vi "ISEG_HVSystemGUI.panel.vi"(0 "object ref":refnum<vi>, 5 "error in (no error)":errorcluster) -> (19 "error out":errorcluster)   [LabVIEW 2014, in "ISEG_HVSystemGUI.lvlib"]
doc: "This is just an example for a ISEG HV System GUI .\n\nLicense Agreement for this software:\n\nCopyright (C)\nGesellschaft für Schwerionenforschung, GSI\nPlanckstr. 1\n64291 Darmstadt\nGermany\n\nContact: D.Beck@gsi.de \n\nThis program is free software; you can redistribute it and/or modify it under the terms of the GNU General Public License as published by the Free Software Foundation; either version 2 of the license, or (at your option) any later version.\n\nThis program is distributed in the hope that it will be useful, but WITHOUT ANYW ARRANTY; without even the implied warranty of MERCHANTABILITY or FITNESS FOR A PARTICULAR PURPOSE. See the GNU General License for more details (http://www.gnu.org).\n\nGesellschaft für Schwerionenforschung, GSI\nPlanckstr. 1, 64291 Darmstadt, Germany\nFor all questions and ideas contact: M.Richter@gsi.de, H.Brand@gsi.de or D.Beck@gsi.de.\nLast update: 18-DEC-2002"
uses:
  ISEG_HVSystemGUI.lvlib
  CSlibraries-extern/DimLVEvent/DimIndicators/DimIndicators.anyType.ctl
  CSlibraries-extern/DimLVEvent/DimIndicators/DimIndicators.numericType.ctl
  CS_Core/CSSystem/CoreDefs/CoreDefs.call_type.ctl
  CS_Core/BaseProcess/BaseProcess.descriptor string definition.ctl
  CS_Core/CSSystem/CoreDefs/CoreDefs.rawDataType.ctl
  CS_Core/CSSystem/CoreLib/CoreLib.short 2 byte array.vi
  CS_Core/CSSystem/CoreLib/CoreLib.double 2 byte array.vi
  CS_Core/CSSystem/CoreLib/CoreLib.string 2 byte array.vi
  CSlibraries/UtilityLib/UtilityLib.lvlib
  CS_Core/CSSystem/CoreLib/CoreLib.lvlib
  CSlibraries-extern/DimLVEvent/DimIndicators/DimIndicators.lvlib
  CS_Core/CSSystem/CSSystemLib/CSSystemLib.lvlib
  CS_Core/BaseProcess/BaseProcess.lvlib
panel:
  in  "Refresh":T1
  in  "Force":T2
  in  "Mode1/Mode2":bool caption="Status_Force"
  in  "Refresh":dbl
  in  "Connected":T2
  in  "Active":T2
  out "Connected":bool
  out "Active":bool
  in  "call cluster in":T3={"Object"="", "Selector"="", "CallType"=enum."synchronous", "Async Object"="", "Async Selector"="", "Data Descriptor"="", "Data"=[], "Error #"=0, "Expire"=0}
  in  "DeviceState":T1
  out "Object Name":string
  in  "Pr ID":T2
  in  "OPC Version":T2
  in  "CAN":T2
  in  "Open BoardGUI":bool
  in  "Board":i16
  in  "stop":bool
  out "Pr ID":string
  out "OPC Version":string
  out "CAN":string caption="Status_CAN bus"
  out "loop counter":i32
  out "time stamp":timestamp
  # ":"
  # "Mode 2"
  # "Mode1"
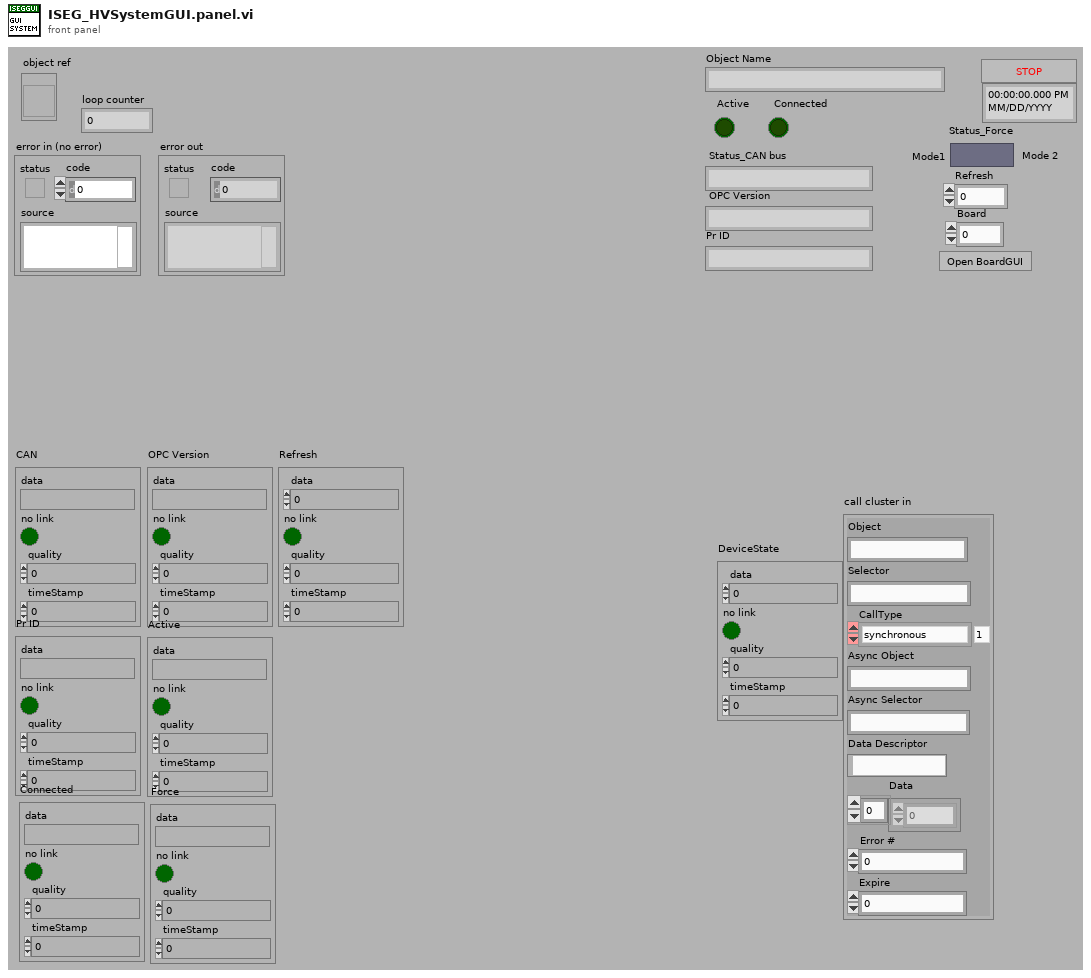
[diagram p1: front panel]
types:
  T1 = typedef "DimIndicators.lvlib/DimIndicators.numericType.ctl" = cluster{"data":dbl, "no link":bool, "quality":i32, "timeStamp":dbl}
  T2 = typedef "DimIndicators.lvlib/DimIndicators.anyType.ctl" = cluster{"data":string, "no link":bool, "quality":i32, "timeStamp":dbl}
  T3 = typedef "CoreDefs.call_type.ctl" = cluster{"Object":string, "Selector":string, "CallType":enum16{"simple", "synchronous", "asynchronous"}, "Async Object":string, "Async Selector":string, "Data Descriptor":T4, "Data":T5, "Error #":i32, "Expire":u32}
  T4 = typedef "BaseProcess.lvlib/BaseProcess.descriptor string definition.ctl" = string
  T5 = typedef "CoreDefs.rawDataType.ctl" = i8[]
  T6 = typedef "ISEG_HVSystemGUI.lvlib/ISEG_HVSystemGUI.i attribute.ctl" = cluster{"System Name":string, "Object Name":string, "Prefix":string}
  T7 = typedef "UtilityLib.lvlib/UtilityLib.valueStatus.ctl" = enum16{"no info available", "stand by/off", "on", "warning", "alarm/malfunction", "not implemented", "user action required", "important information", "system default", "control default", "indicator default", "button default"}
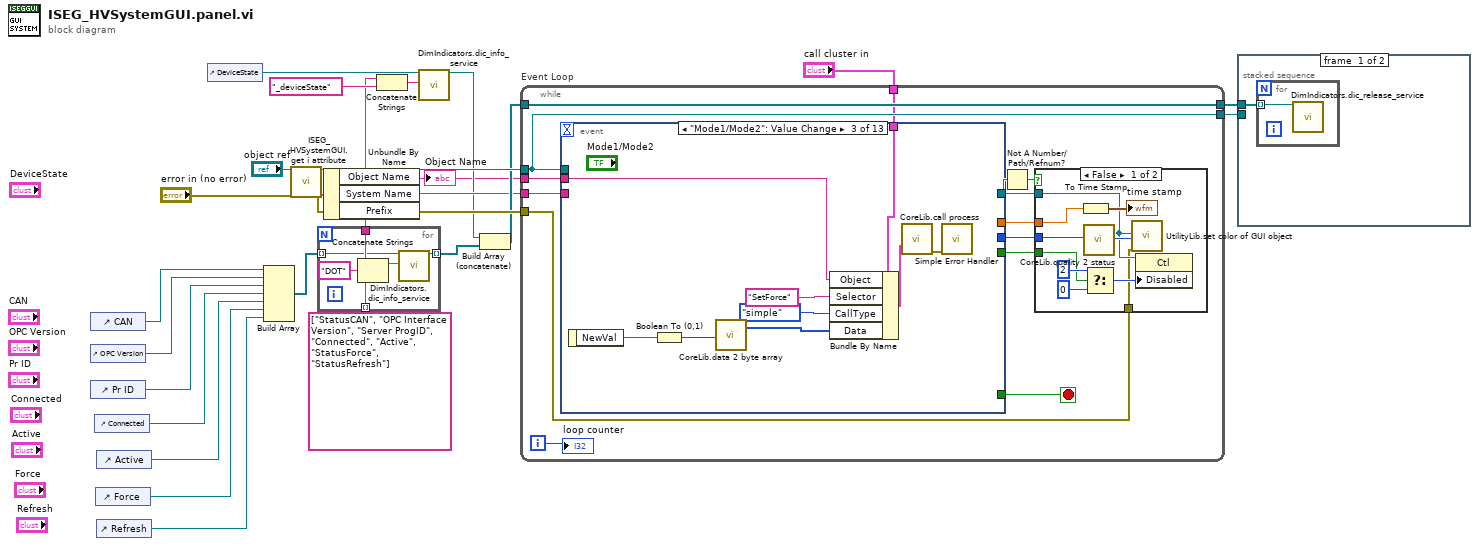
[diagram p0: block diagram]
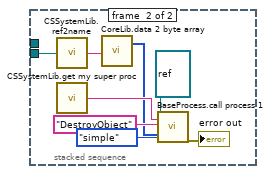
[diagram p2: hidden frame]
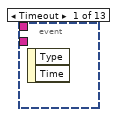
[diagram p4: hidden frame]
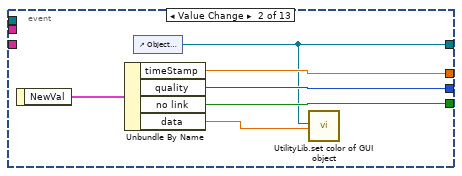
[diagram p5: hidden frame]
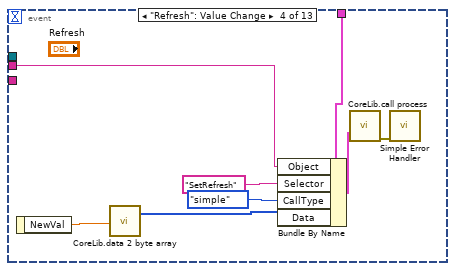
[diagram p6: hidden frame]
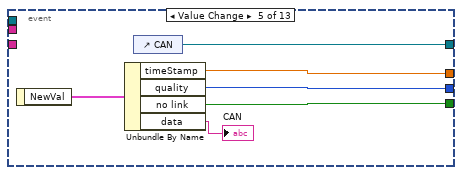
[diagram p7: hidden frame]
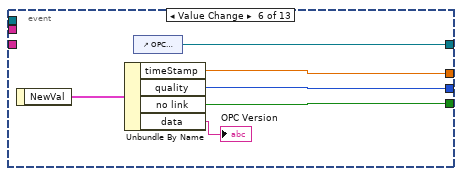
[diagram p8: hidden frame]
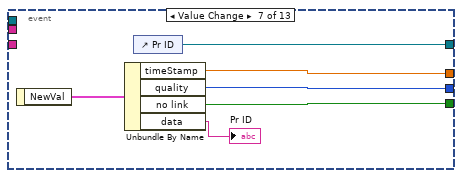
[diagram p9: hidden frame]
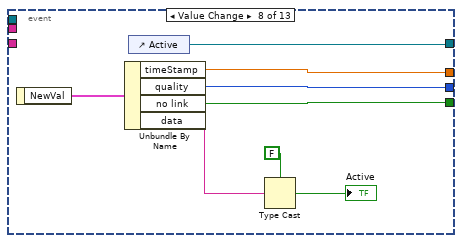
[diagram p10: hidden frame]
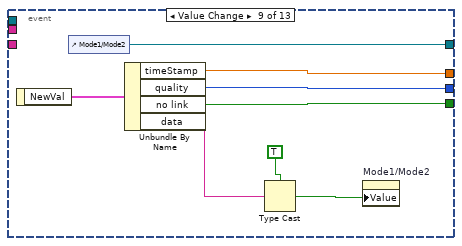
[diagram p11: hidden frame]
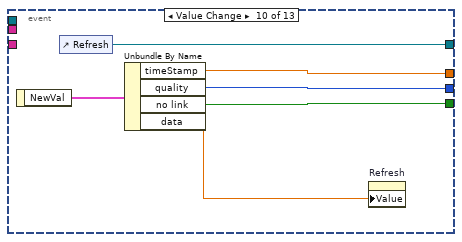
[diagram p12: hidden frame]
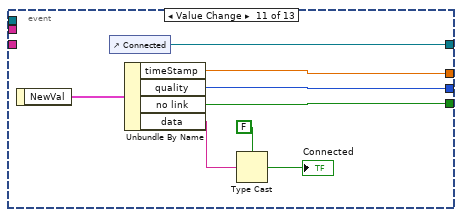
[diagram p13: hidden frame]
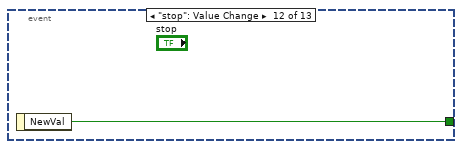
[diagram p14: hidden frame]
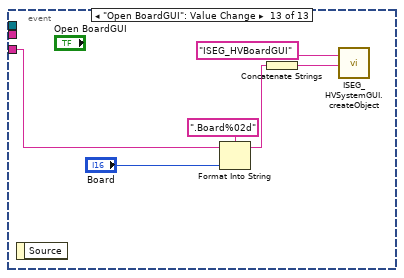
[diagram p15: hidden frame]
diagram:
  n1 = control-ref of="CAN"() -> (w9:refnum<vi>)
  n2 = control-ref of="OPC Version"() -> (w8:refnum<vi>)
  n3 = control-ref of="Pr ID"() -> (w7:refnum<vi>)
  n4 = control-ref of="Connected"() -> (w3:refnum<vi>)
  n5 = control-ref of="Force"() -> (w2:refnum<vi>)
  n6 = control-ref of="Active"() -> (w4:refnum<vi>)
  n7 = control-ref of="Refresh"() -> (w1:refnum<vi>)
  n8 = control-ref of="DeviceState"() -> (w12:refnum<vi>)
  n9 = Build Array(w9, w8, w7, w3, w4, w2, w1) -> (w21:refnum<vi>[])
  n10 = call "ISEG_HVSystemGUI.get i attribute.vi"("i ref in"="object ref", "error in (no error)"="error in (no error)") -> ("i ref out"=w24:refnum<vi>, "i attribute"=w23:T6, "error out"=w18:errorcluster)  [unwired: 15 in]
  n11 = Unbundle By Name(w23) -> ("Object Name"=w11:string, "System Name"=w16:string, "Prefix"=w5:string)
  "Object Name" <- w11
  n12 = for {
    tunnel: w5 -> [w31]
    tunnel: string[] ["StatusCAN", "OPC Interface Version", "Server ProgID", "Connected", "Active", "StatusForce", "StatusRefresh"] ("Properties") -> [w30] mode=indexing
    tunnel: w21 -> [w28] mode=indexing
    tunnel: [w27] -> w6 mode=indexing
    n13 = Concatenate Strings(w31, "DOT" ("string"), w30) -> (w29:string)
    n14 = call "DimIndicators.dic_info_service.vi"("controlRef"=w28, "serviceName"=w29) -> ("controlRef out"=w27:refnum<vi>)  [unwired: 16 in, 1 out]
  }
  n15 = Concatenate Strings(w11, "_deviceState" ("string")) -> (w14:string)
  n16 = call "DimIndicators.dic_info_service.vi"("controlRef"=w12, "serviceName"=w14) -> ("controlRef out"=w13:refnum<vi>)  [unwired: 16 in, 1 out]
  n17 = Build Array (concatenate)(w13, w6) -> (w17:refnum<vi>[])
  n18 = while "Event Loop" {
    tunnel: w24 -> [w43]
    tunnel: [w43] -> w26
    tunnel: [w42] -> w20
    tunnel: w17 -> [w42]
    tunnel: w18 -> [w39]
    tunnel: w16 -> [w38]
    tunnel: w11 -> [w34]
    tunnel: "call cluster in" -> [w33]
    i -> [w44]
    stop <- w45 stop-if-true
    n19 = event shown="[2] \"Mode1/Mode2\": Value Change" {
      selector: _ -> [_ _ _ _ _ _ _ _ _ _ _ _ _]
      dyn-events: _ -> [_ _ _ _ _ _ _ _ _ _ _ _ _]
      timeout: _ -> [_ _ _ _ _ _ _ _ _ _ _ _ _]
      tunnel: [_ _ _ _ _ _ _ _ _ _ _ w127 _] -> w45
      tunnel: w43 -> [_ _ _ _ _ _ _ _ _ _ _ _ _]
      tunnel: [_ w60 _ _ w84 w90 w96 w104 w112 w118 w126 _ _] -> w41
      tunnel: [_ w59 _ _ w83 w89 w95 w103 w111 w117 w125 _ _] -> w40
      tunnel: [_ w57 _ _ w82 w88 w94 w100 w107 w114 w122 _ _] -> w35
      tunnel: [_ w58 _ _ w81 w87 w93 w102 w110 w116 w124 _ _] -> w37
      tunnel: w38 -> [_ _ _ _ _ _ _ _ _ _ _ _ w133]
      tunnel: w34 -> [_ _ w65 w74 _ _ _ _ _ _ _ _ _]
      tunnel: w33 -> [_ _ w66 w75 _ _ _ _ _ _ _ _ _]
      event Timeout {
        n20 = event-data() -> ()  [unwired: 1 in, 2 out]
      }
      event Value Change {
        n21 = event-data() -> ("NewVal"=w61:T1)  [unwired: 1 in]
        n22 = Unbundle By Name(w61) -> ("timeStamp"=w58:dbl, "quality"=w60:i32, "no link"=w59:bool, "data"=w56:dbl)
        n23 = control-ref of="Object Name"() -> (w57:refnum<vi>)
        n24 = call "UtilityLib.set color of GUI object.vi"("GUI object Ref"=w57, "valueStatus"=w56) -> ()  [unwired: 17 in, 1 out]
      }
      event "Mode1/Mode2": Value Change {
        n25 = event-data() -> ("NewVal"=w67:bool)  [unwired: 1 in]
        n26 = Boolean To (0,1)(Boolean=w67) -> (0, 1=w63:i16)
        n27 = call-poly "CoreLib.data 2 byte array.vi"("i16"=w63) -> ("byteArray out"=w62:T5)  [unwired: 18 in]
        n28 = Bundle By Name(cluster=w66, "Object"=w65, "Selector"="SetForce", "CallType"=enum16{"simple", "synchronous", "asynchronous"}."simple", "Data"=w62) -> (w64:T3)
        n29 = call "CoreLib.call process.vi"("call cluster in"=w64) -> ("error out"=w70:errorcluster)  [unwired: 13 in, 1 out]
        n30 = call <vilib>:"Simple Error Handler.vi"("error in (no error)"=w70) -> ()  [unwired: 4 in, 5 out]
      }
      event "Refresh": Value Change {
        n31 = event-data() -> ("NewVal"=w71:dbl)  [unwired: 1 in]
        n32 = call-poly "CoreLib.data 2 byte array.vi"("f64"=w71) -> ("byteArray out"=w72:T5)  [unwired: 18 in]
        n33 = Bundle By Name(cluster=w75, "Object"=w74, "Selector"="SetRefresh", "CallType"=enum16{"simple", "synchronous", "asynchronous"}."simple", "Data"=w72) -> (w73:T3)
        n34 = call "CoreLib.call process.vi"("call cluster in"=w73) -> ("error out"=w78:errorcluster)  [unwired: 13 in, 1 out]
        n35 = call <vilib>:"Simple Error Handler.vi"("error in (no error)"=w78) -> ()  [unwired: 4 in, 5 out]
      }
      event Value Change {
        n36 = event-data() -> ("NewVal"=w80:T2)  [unwired: 1 in]
        n37 = Unbundle By Name(w80) -> ("timeStamp"=w81:dbl, "quality"=w84:i32, "no link"=w83:bool, "data"=→"CAN":string)
        n38 = control-ref of="CAN"() -> (w82:refnum<vi>)
      }
      event Value Change {
        n39 = event-data() -> ("NewVal"=w86:T2)  [unwired: 1 in]
        n40 = Unbundle By Name(w86) -> ("timeStamp"=w87:dbl, "quality"=w90:i32, "no link"=w89:bool, "data"=→"OPC Version":string)
        n41 = control-ref of="OPC Version"() -> (w88:refnum<vi>)
      }
      event Value Change {
        n42 = event-data() -> ("NewVal"=w92:T2)  [unwired: 1 in]
        n43 = Unbundle By Name(w92) -> ("timeStamp"=w93:dbl, "quality"=w96:i32, "no link"=w95:bool, "data"=→"Pr ID":string)
        n44 = control-ref of="Pr ID"() -> (w94:refnum<vi>)
      }
      event Value Change {
        n45 = event-data() -> ("NewVal"=w101:T2)  [unwired: 1 in]
        n46 = Unbundle By Name(w101) -> ("timeStamp"=w102:dbl, "quality"=w104:i32, "no link"=w103:bool, "data"=w99:string)
        n47 = control-ref of="Active"() -> (w100:refnum<vi>)
        n48 = Type Cast(type=FALSE, x=w99) -> (*(type *) &x=→"Active":bool)
      }
      event Value Change {
        n49 = event-data() -> ("NewVal"=w108:T2)  [unwired: 1 in]
        n50 = control-ref of="Mode1/Mode2"() -> (w107:refnum<vi>)
        n51 = Unbundle By Name(w108) -> ("timeStamp"=w110:dbl, "quality"=w112:i32, "no link"=w111:bool, "data"=w109:string)
        n52 = Type Cast(type=TRUE, x=w109) -> (*(type *) &x=w105:bool)
        n53 = property on="Mode1/Mode2" class="Bool (strict)"("Value"=w105) -> ()  [unwired: 2 in, 2 out]
      }
      event Value Change {
        n54 = event-data() -> ("NewVal"=w115:T1)  [unwired: 1 in]
        n55 = control-ref of="Refresh"() -> (w114:refnum<vi>)
        n56 = Unbundle By Name(w115) -> ("timeStamp"=w116:dbl, "quality"=w118:i32, "no link"=w117:bool, "data"=w113:dbl)
        n57 = property on="Refresh" class="DigNum (strict)"("Value"=w113) -> ()  [unwired: 2 in, 2 out]
      }
      event Value Change {
        n58 = event-data() -> ("NewVal"=w123:T2)  [unwired: 1 in]
        n59 = control-ref of="Connected"() -> (w122:refnum<vi>)
        n60 = Unbundle By Name(w123) -> ("timeStamp"=w124:dbl, "quality"=w126:i32, "no link"=w125:bool, "data"=w119:string)
        n61 = Type Cast(type=FALSE, x=w119) -> (*(type *) &x=→"Connected":bool)
      }
      event "stop": Value Change {
        n62 = event-data() -> ("NewVal"=w127:bool)  [unwired: 1 in]
      }
      event "Open BoardGUI": Value Change {
        n63 = event-data() -> ()  [unwired: 1 in, 1 out]
        n64 = Format Into String(format string=".Board%02d", initial string=w133, "Board") -> (resulting string=w128:string)  [unwired: 1 in, 1 out]
        n65 = Concatenate Strings(w128) -> (w130:string)
        n66 = call "ISEG_HVSystemGUI.createObject.vi"("Class name"="ISEG_HVBoardGUI" ("class name"), "data"=w130) -> ()  [unwired: 17 in, 1 out]
      }
    }
    n67 = Not A Number/Path/Refnum?(number/path/refnum=w35) -> (NaN/Path/Refnum?=w36:bool)
    n68 = case shown="False" w36 {
      tunnel: w41 -> [w52 _]
      tunnel: w40 -> [w51 _]
      tunnel: w35 -> [w47 _]
      tunnel: w37 -> [w49 _]
      tunnel: w39 -> [w46 _]
      frame False {
        n69 = To Time Stamp(1:w49) -> (0:→"time stamp":timestamp)
        n70 = call "CoreLib.quality 2 status.vi"("quality"=w52) -> ("valueStatus"=w48:T7)  [unwired: 18 in]
        n71 = Select(t=u8 2 ("Disabled"), s=w51, f=u8 0) -> (s? t:f=w55:u8)
        n72 = call "UtilityLib.set color of GUI object.vi"("GUI object Ref"=w47, "valueStatus"=w48, "error in (no error)"=w46) -> ()  [unwired: 16 in, 1 out]
        n73 = property class="Ctl"(reference=w47, "Disabled"=w55) -> ()  [unwired: 1 in, 2 out]
      }
      frame True {
      }
    }
    "loop counter" <- w44
  }
  n74 = stacked-sequence {
    tunnel: w26 -> [_ w137]
    tunnel: w20 -> [w134 _]
    frame #0 {
      n75 = for {
        tunnel: w134 -> [w135] mode=indexing
        n76 = call "DimIndicators.dic_release_service.vi"("controlRef"=w135) -> ()  [unwired: 18 in, 1 out]
      }
    }
    frame #1 {
      n77 = call "CSSystemLib.ref2name.vi"("obj refnum"=w137) -> ("name"=w141:string)
      n78 = call "CSSystemLib.get my super proc.vi"() -> ("name"=w142:string)  [unwired: 1 in]
      n79 = call-poly "CoreLib.data 2 byte array.vi"("string"=w141) -> ("byteArray out"=w139:T5)  [unwired: 18 in]
      n80 = call "BaseProcess.call process 1.vi"("i ref in"=refnum<vi> refnum, "Object"=w142, "Selector"="DestroyObject", "CallType"=enum16{"simple", "synchronous", "asynchronous"}."simple", "Data"=w139) -> ("error out"=→"error out":errorcluster)  [unwired: 12 in, 2 out]
    }
  }
